vi "Prepare Logging Loop.vi"(8 "error in (no error)":errorcluster, 10 "Tweezertron Ctrl Refs":T1, 11 "Queue in":refnum<queue>) -> (0 "error out":errorcluster, 2 "Tweezertron Ctrl Refs out":T1, 3 "Queue out":refnum<queue>)   [LabVIEW 2020]
uses:
  _Controls/Logging Queue Cluster.ctl
  _Controls/Tweezertron Ctrl Refs.ctl
  _Controls/Confocal Controls.ctl
  _Controls/iFlex.ctl
  _Controls/PIFOC Position.ctl
  _Controls/Manlight Controls.ctl
  _Controls/Exp Params.ctl
  _Controls/Image Thresholds.ctl
  _Controls/Spots.ctl
  _Controls/Spot Params.ctl
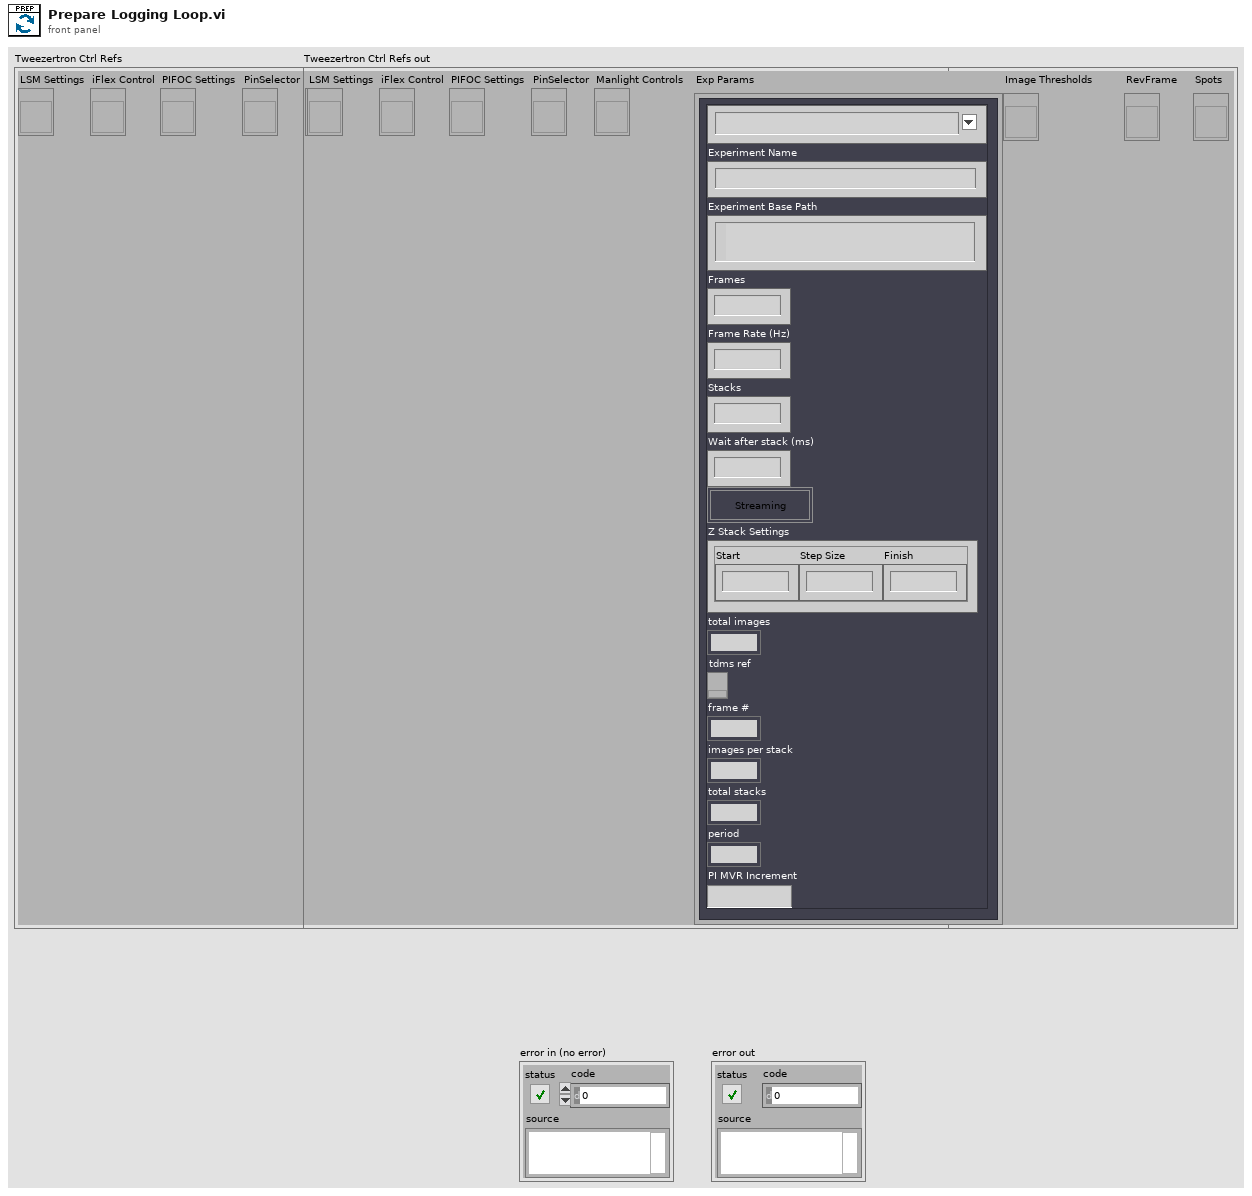
[diagram p1: front panel]
types:
  T1 = typedef "Tweezertron Ctrl Refs.ctl" = cluster{"LSM Settings":refnum<vi>, "iFlex Control":refnum<vi>, "PIFOC Settings":refnum<vi>, "PinSelector":refnum<vi>, "Manlight Controls":refnum<vi>, "Exp Params":refnum<vi>, "Image Thresholds":refnum<vi>, "RevFrame":refnum<vi>, "Spots":refnum<vi>}
  T2 = typedef "Logging Queue Cluster.ctl" = cluster{"message":string, "Data for Logging":cluster{"pDataBuffer":u16[], "timestamp (ns)":u64, "PI pos (um)":dbl}, "Tweezertron Ctrl Refs":T1}
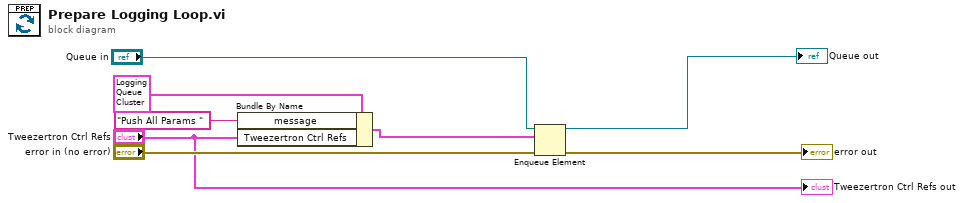
[diagram p0: block diagram]
diagram:
  n1 = Bundle By Name(cluster=T2 {"message"="", "Data for Logging"={"pDataBuffer"=[], "timestamp (ns)"=0, "PI pos (um)"=0.0}, "Tweezertron Ctrl Refs"={"LSM Settings"=refnum, "iFlex Control"=refnum, "PIFOC Settings"=refnum, "PinSelector"=refnum, "Manlight Controls"=refnum, "Exp Params"=refnum, "Image Thresholds"=refnum, "RevFrame"=refnum, "Spots"=refnum}} ("Logging Queue Cluster"), "message"="Push All Params ", "Tweezertron Ctrl Refs"="Tweezertron Ctrl Refs") -> (w3:T2)
  n2 = Enqueue Element(queue="Queue in", element=w3, error in (no error)="error in (no error)") -> (queue out=→"Queue out":refnum<queue>, error out=→"error out":errorcluster)  [unwired: 1 in, 1 out]
  "Tweezertron Ctrl Refs out" <- "Tweezertron Ctrl Refs"
